vi "test_libssh2_session_handshake.vi"() -> ()   [LabVIEW 2013, in "libssh2_integration_tests.lvlib"]
uses:
  libssh2_integration_tests.lvlib
  libssh2/libssh2_init_default.vi
  libssh2/libssh2_session_handshake_tcp.vi
  <vilib>/addons/_JKI Toolkits/Caraya/classes/Assert/Assert Not Error.vi
  <vilib>/addons/_JKI Toolkits/Caraya/classes/Test/Test.lvclass
  <vilib>/addons/_JKI Toolkits/Caraya/classes/Assert/Assert.lvclass
  libssh2/libssh2.lvlib
panel:
  out "error out":errorcluster
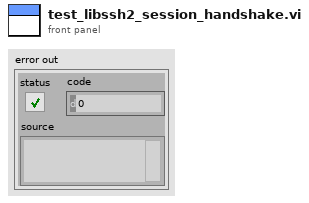
[diagram p1: front panel]
types:
  T1 = typedef "libssh2.lvlib/Session Refnum.ctl" = refnum<k1>
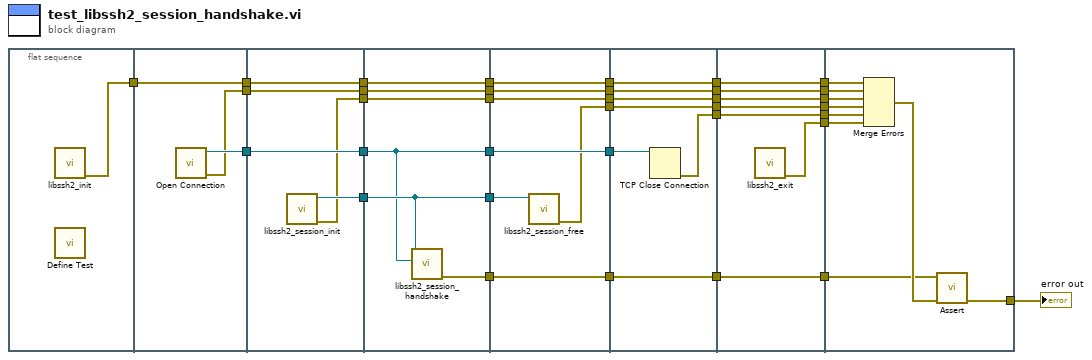
[diagram p0: block diagram]
diagram:
  n1 = flat-sequence {
    tunnel: [w36] -> w35
    tunnel: [w39] -> w27
    tunnel: w35 -> [w38]
    tunnel: [w38] -> w26
    tunnel: [w37] -> w25
    tunnel: w27 -> [w44]
    tunnel: [w44] -> w24
    tunnel: w26 -> [w43]
    tunnel: [w43] -> w23
    tunnel: w25 -> [w42]
    tunnel: [w42] -> w22
    tunnel: [w41] -> w14
    tunnel: [w40] -> w13
    tunnel: w24 -> [w45]
    tunnel: [w45] -> w21
    tunnel: w23 -> [w50]
    tunnel: [w50] -> w19
    tunnel: w22 -> [w49]
    tunnel: [w49] -> w17
    tunnel: [w48] -> w15
    tunnel: w14 -> [w48]
    tunnel: w13 -> [w47]
    tunnel: [w47] -> w12
    tunnel: [w46] -> w5
    tunnel: w21 -> [w57]
    tunnel: [w57] -> w20
    tunnel: w19 -> [w56]
    tunnel: [w56] -> w18
    tunnel: w17 -> [w55]
    tunnel: [w55] -> w16
    tunnel: w15 -> [w54]
    tunnel: w12 -> [w53]
    tunnel: [w53] -> w11
    tunnel: [w52] -> w8
    tunnel: w5 -> [w51]
    tunnel: [w51] -> w4
    tunnel: w20 -> [w64]
    tunnel: w18 -> [w63]
    tunnel: [w63] -> w34
    tunnel: w16 -> [w62]
    tunnel: [w62] -> w32
    tunnel: [w61] -> w30
    tunnel: w11 -> [w60]
    tunnel: [w60] -> w10
    tunnel: w8 -> [w59]
    tunnel: [w59] -> w7
    tunnel: w4 -> [w58]
    tunnel: [w58] -> w3
    tunnel: w34 -> [w71]
    tunnel: [w71] -> w33
    tunnel: w32 -> [w70]
    tunnel: [w70] -> w31
    tunnel: w30 -> [w69]
    tunnel: [w69] -> w29
    tunnel: [w68] -> w28
    tunnel: w10 -> [w67]
    tunnel: [w67] -> w9
    tunnel: w7 -> [w66]
    tunnel: [w66] -> w6
    tunnel: w3 -> [w65]
    tunnel: [w65] -> w2
    tunnel: w33 -> [w80]
    tunnel: w31 -> [w79]
    tunnel: w29 -> [w78]
    tunnel: w28 -> [w77]
    tunnel: w9 -> [w76]
    tunnel: w6 -> [w75]
    tunnel: w2 -> [w73]
    tunnel: [w72] -> w1
    frame #0 {
      n2 = call-poly "libssh2_init.vi"() -> ("error out"=w36:errorcluster)  [unwired: 11 in]
      n3 = call <vilib>:"Define Test.vi"() -> ()  [unwired: 10 in, 2 out]
    }
    frame #1 {
      n4 = call "Open Connection.vi"() -> ("error out"=w37:errorcluster, "connection ID"=w39:refnum<k5>)  [unwired: 10 in]
    }
    frame #2 {
      n5 = call "libssh2_session_init.vi"() -> ("error out"=w40:errorcluster, "session"=w41:T1)  [unwired: 10 in]
    }
    frame #3 {
      n6 = call-poly "libssh2_session_handshake.vi"("tcp connection"=w45, "session"=w48) -> ("error out"=w46:errorcluster)  [unwired: 9 in]
    }
    frame #4 {
      n7 = call "libssh2_session_free.vi"("session"=w54) -> ("error out"=w52:errorcluster)  [unwired: 10 in]
    }
    frame #5 {
      n8 = TCP Close Connection(connection ID=w64) -> (error out=w61:errorcluster)  [unwired: 2 in, 1 out]
    }
    frame #6 {
      n9 = call "libssh2_exit.vi"() -> ("error out"=w68:errorcluster)  [unwired: 11 in]
    }
    frame #7 {
      n10 = Merge Errors(w80, w79, w76, w75, w78, w77) -> (w74:errorcluster)
      n11 = call-poly <vilib>:"Assert.vi"("error in (no error)"=w74, "Not Error?"=w73) -> ("error out"=w72:errorcluster)  [unwired: 8 in, 1 out]
    }
  }
  "error out" <- w1
